vi "Dereference Outline Glyph.vi"(8 "error in (no error)":errorcluster, 11 "glyph ref in":i64) -> (0 "error out":errorcluster, 2 "Outline Glyph Rec":T1, 3 "glyph ref out":i64)   [LabVIEW 2023, in "Freetype Drawer.lvlib"]
uses:
  Freetype Drawer.lvlib
  Outline Glyph Rec.ctl
  Glyph Rec.ctl
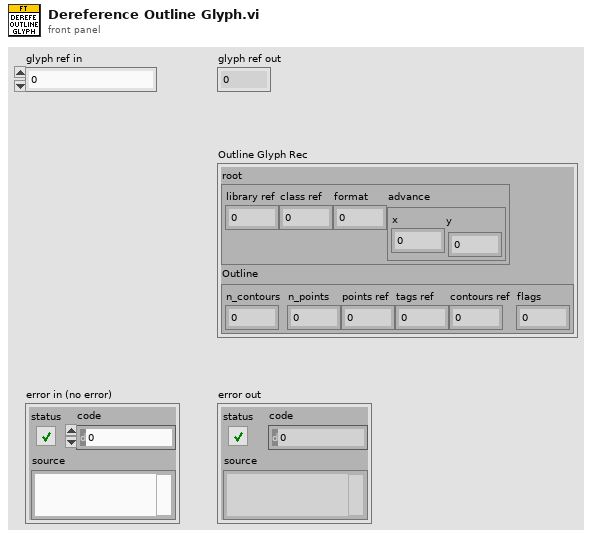
[diagram p1: front panel]
types:
  T1 = typedef "Freetype Drawer.lvlib/Outline Glyph Rec.ctl" = cluster{"root":T2, "Outline":cluster{"n_contours":i16, "n_points":i16, "points ref":i64, "tags ref":i64, "contours ref":i64, "flags":i32}}
  T2 = typedef "Freetype Drawer.lvlib/Glyph Rec.ctl" = cluster{"library ref":i64, "class ref":i64, "format":i32, "advance":cluster{"x":i32, "y":i32}}
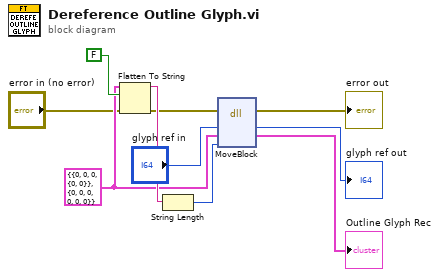
[diagram p0: block diagram]
diagram:
  w7 = T1 {"root"={"library ref"=0, "class ref"=0, "format"=0, "advance"={"x"=0, "y"=0}}, "Outline"={"n_contours"=0, "n_points"=0, "points ref"=0, "tags ref"=0, "contours ref"=0, "flags"=0}} ("Outline Glyph Rec")
  n1 = Flatten To String(anything=w7, prepend array or string size? (T)=FALSE, error in (no error)="error in (no error)") -> (data string=w9:string, error out=w3:errorcluster)  [unwired: 1 in, 1 out]
  n2 = String Length(string=w9) -> (length=w2:i32)
  n3 = dll-call lib="LabVIEW" fn="MoveBlock"(error in=w3, "in"="glyph ref in", "out"=w7, "size"=w2) -> (error out=→"error out":errorcluster, "in"=→"glyph ref out":i64, "out"=→"Outline Glyph Rec":T1)  [unwired: 4 in, 1 out]
